vi "Egi1_Pitch_Roll_Angel_Set_Get.vi"(0 "Egi1 Roll Angle":dbl, 1 "Egi1 Roll Angle Valid":u16, 2 "message handle in 2":u64, 3 "message handle in1":u64, 5 "error in (no error)":errorcluster, 6 "Egi1 Pitch Angle Valid":u16, 8 "Egi1 Pitch Angle":dbl) -> (9 "Egi1 Roll Angle Range Message":string, 10 "Egi1 Pitch Angle Range Message":string, 11 "Egi1 Roll Angle Value NEW":u32 format="%08x", 14 "Egi1 Pitch Angle Value OLD":u32 format="%.0x", 16 "Egi1 Pitch Angle Value NEW":u32 format="%08x", 17 "Egi1 Roll Angle Value OLD":u32 format="%.0x", 19 "error out":errorcluster)   [LabVIEW 2023]
uses:
  <instrlib>/BTI429Lib/Private/Utility/Get BNR Data.vi
  <instrlib>/BTI429Lib/Private/Utility/Set BNR Data.vi
  <instrlib>/BTI429Lib/Private/Utility/Set BNR SSM.vi
  <instrlib>/BTI429Lib/BTI429LV.lvlib
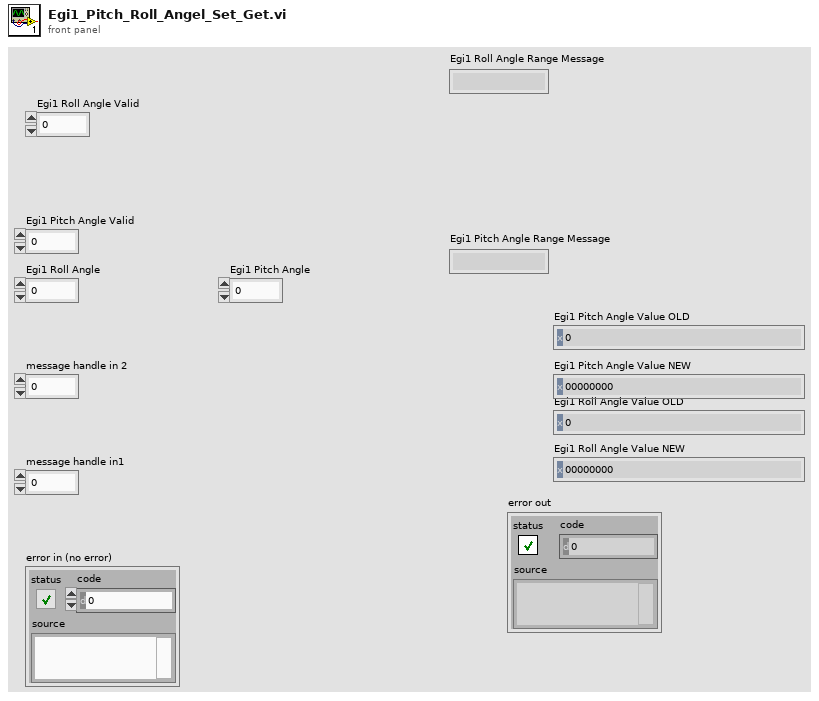
[diagram p1: front panel]
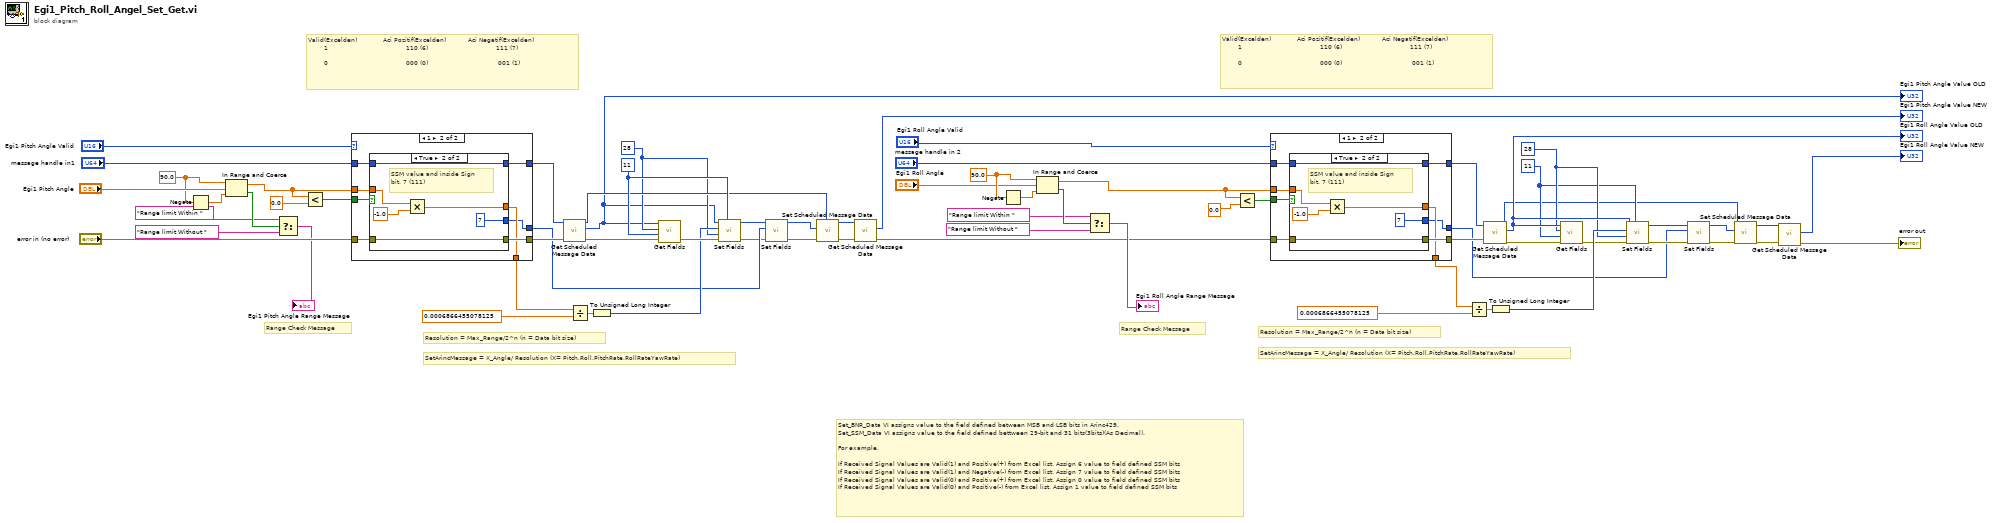
[diagram p0: block diagram]
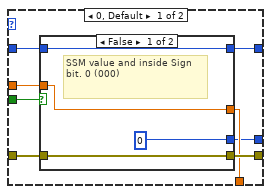
[diagram p2: hidden frame]
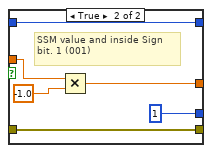
[diagram p3: hidden frame]
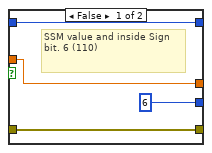
[diagram p4: hidden frame]
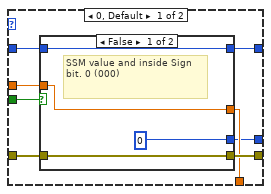
[diagram p5: hidden frame]
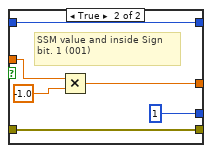
[diagram p6: hidden frame]
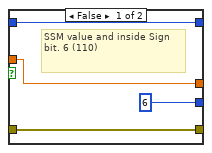
[diagram p7: hidden frame]
diagram:
  w34 = 90.0 ("upper limit")
  w40 = 90.0 ("upper limit")
  w52 = u16 28 ("most significant bit")
  w51 = u16 11 ("least significant bit")
  w23 = u16 28 ("most significant bit")
  w43 = u16 11 ("least significant bit")
  # "Range Check Message"
  # "Range Check Message"
  # "SetArincMessage = X_Angle/ Resolution (X= Pitch,Roll,PitchRate,RollRateYawRate)"
  # "Resolution = Max_Range/2^n (n = Data bit size)"
  # "SetArincMessage = X_Angle/ Resolution (X= Pitch,Roll,PitchRate,RollRateYawRate)"
  # "Resolution = Max_Range/2^n (n = Data bit size)"
  # "Set_BNR_Data VI assigns value to the field defined between MSB and LSB bits in Arinc429.\nSet_SSM_Data VI assigns value to the field defined bettween 29-bit and 31 bits(3bits)(As Decimal).\n\nFor example,\n\nIf Received Signal Values are Valid(1) and Positive(+) from Excel list. Assign 6 value to field defined SSM bits\nIf Received Signal Values are Valid(1) and Negative(-) from Excel list. Assign 7 value to field defined SSM bits\nIf Received Signal Values are Valid(0) and Positive(+) from Excel list. Assign 0 value to field defined SSM bits\nIf Received Signal Values are Valid(0) and Positive(-) from Excel list. Assign 1 value to field defined SSM bits"
  # "Valid(Excelden)             Aci Pozitif(Excelden)           Aci Negatif(Excelden) \n        1                                       110 (6)                                  111 (7)\n\n        0                                       000 (0)                                   001 (1)"
  # "Valid(Excelden)             Aci Pozitif(Excelden)           Aci Negatif(Excelden) \n        1                                       110 (6)                                  111 (7)\n\n        0                                       000 (0)                                   001 (1)"
  n1 = Negate(x=w40) -> (-x=w39:dbl)
  n2 = In Range and Coerce(upper limit=w40, x="Egi1 Pitch Angle", lower limit=w39) -> (coerced(x)=w21:dbl, In Range?=w38:bool)
  n3 = Select(t="Range limit Within ", s=w38, f="Range limit Without ") -> (s? t:f=→"Egi1 Pitch Angle Range Message":string)
  n4 = Less?(x=w21, y=0.0) -> (x < y?=w46:bool)
  n5 = case shown="1" "Egi1 Pitch Angle Valid" {
    tunnel: [w74 w93] -> w56
    tunnel: [w72 w92] -> w55
    tunnel: "error in (no error)" -> [w75 w91]
    tunnel: "message handle in1" -> [w73 w90]
    tunnel: w46 -> [w70 w89]
    tunnel: [w69 w88] -> w27
    tunnel: w21 -> [w71 w87]
    tunnel: [w68 w86] -> w19
    frame 0, Default {
      n6 = case shown="False" w70 {
        tunnel: w71 -> [w79 w81]
        tunnel: [w79 w84] -> w69
        tunnel: w73 -> [w78 w83]
        tunnel: w75 -> [w77 w82]
        tunnel: [w78 w83] -> w72
        tunnel: [w77 w82] -> w74
        tunnel: [u16 0 ("value") u16 1 ("value")] -> w68
        frame False {
          # "SSM value and inside Sign bit. 0 (000)"
        }
        frame True {
          # "SSM value and inside Sign bit. 1 (001)"
          n7 = Multiply(x=w81, y=-1.0) -> (x*y=w84:dbl)
        }
      }
    }
    frame 1 {
      n8 = case shown="True" w89 {
        tunnel: w87 -> [w97 w102]
        tunnel: [w97 w101] -> w88
        tunnel: w90 -> [w96 w100]
        tunnel: w91 -> [w95 w99]
        tunnel: [w96 w100] -> w92
        tunnel: [w95 w99] -> w93
        tunnel: [u16 6 ("value") u16 7 ("value")] -> w86
        frame False {
          # "SSM value and inside Sign bit. 6 (110)"
        }
        frame True {
          # "SSM value and inside Sign bit. 7 (111)"
          n9 = Multiply(x=w102, y=-1.0) -> (x*y=w101:dbl)
        }
      }
    }
  }
  n10 = call <instrlib>:"Get Scheduled Message Data.vi"("error in (no error)"=w56, "message handle in"=w55) -> ("error out"=w22:errorcluster, "value"=w16:u32, "message handle out"=w26:u64)  [unwired: 7 in]
  "Egi1 Pitch Angle Value OLD" <- w16
  n11 = Divide(x=w27, y=0.0006866455078125) -> (x/y=w47:dbl)
  n12 = To Unsigned Long Integer(number=w47) -> (unsigned 32bit integer=w24:u32)
  n13 = call-poly <instrlib>:"Get Fields.vi"("error in (no error)"=w22, "least significant bit"=w43, "most significant bit"=w23, "message"=w16) -> ("error out"=w25:errorcluster)  [unwired: 6 in, 1 out]
  n14 = call-poly <instrlib>:"Set Fields.vi"("least significant bit"=w43, "error in (no error)"=w25, "most significant bit"=w23, "value"=w24, "message"=w16) -> ("error out"=w14:errorcluster, "message out"=w15:u32)  [unwired: 5 in]
  n15 = call-poly <instrlib>:"Set Fields.vi"("error in (no error)"=w14, "value"=w19, "message"=w15) -> ("error out"=w18:errorcluster, "message out"=w17:u32)  [unwired: 7 in]
  n16 = call <instrlib>:"Set Scheduled Message Data.vi"("error in (no error)"=w18, "value"=w17, "message handle in"=w26) -> ("error out"=w65:errorcluster, "message handle out"=w66:u64)  [unwired: 7 in]
  n17 = call <instrlib>:"Get Scheduled Message Data.vi"("error in (no error)"=w65, "message handle in"=w66) -> ("error out"=w13:errorcluster, "value"=→"Egi1 Pitch Angle Value NEW":u32)  [unwired: 7 in, 1 out]
  n18 = Negate(x=w34) -> (-x=w33:dbl)
  n19 = In Range and Coerce(upper limit=w34, x="Egi1 Roll Angle", lower limit=w33) -> (coerced(x)=w8:dbl, In Range?=w32:bool)
  n20 = Select(t="Range limit Within ", s=w32, f="Range limit Without ") -> (s? t:f=→"Egi1 Roll Angle Range Message":string)
  n21 = Less?(x=w8, y=0.0) -> (x < y?=w7:bool)
  n22 = case shown="1" "Egi1 Roll Angle Valid" {
    tunnel: [w110 w129] -> w11
    tunnel: [w106 w128] -> w10
    tunnel: w13 -> [w111 w127]
    tunnel: "message handle in 2" -> [w105 w126]
    tunnel: w7 -> [w104 w125]
    tunnel: [w108 w124] -> w12
    tunnel: w8 -> [w109 w123]
    tunnel: [w107 w122] -> w1
    frame 0, Default {
      n23 = case shown="False" w104 {
        tunnel: w109 -> [w115 w117]
        tunnel: [w115 w120] -> w108
        tunnel: w105 -> [w114 w119]
        tunnel: w111 -> [w113 w118]
        tunnel: [w114 w119] -> w106
        tunnel: [w113 w118] -> w110
        tunnel: [u16 0 ("value") u16 1 ("value")] -> w107
        frame False {
          # "SSM value and inside Sign bit. 0 (000)"
        }
        frame True {
          # "SSM value and inside Sign bit. 1 (001)"
          n24 = Multiply(x=w117, y=-1.0) -> (x*y=w120:dbl)
        }
      }
    }
    frame 1 {
      n25 = case shown="True" w125 {
        tunnel: w123 -> [w133 w138]
        tunnel: [w133 w137] -> w124
        tunnel: w126 -> [w132 w136]
        tunnel: w127 -> [w131 w135]
        tunnel: [w132 w136] -> w128
        tunnel: [w131 w135] -> w129
        tunnel: [u16 6 ("value") u16 7 ("value")] -> w122
        frame False {
          # "SSM value and inside Sign bit. 6 (110)"
        }
        frame True {
          # "SSM value and inside Sign bit. 7 (111)"
          n26 = Multiply(x=w138, y=-1.0) -> (x*y=w137:dbl)
        }
      }
    }
  }
  n27 = Divide(x=w12, y=0.0006866455078125) -> (x/y=w59:dbl)
  n28 = call <instrlib>:"Get Scheduled Message Data.vi"("error in (no error)"=w11, "message handle in"=w10) -> ("error out"=w49:errorcluster, "value"=w61:u32, "message handle out"=w48:u64)  [unwired: 7 in]
  "Egi1 Roll Angle Value OLD" <- w61
  n29 = To Unsigned Long Integer(number=w59) -> (unsigned 32bit integer=w60:u32)
  n30 = call-poly <instrlib>:"Get Fields.vi"("error in (no error)"=w49, "least significant bit"=w51, "most significant bit"=w52, "message"=w61) -> ("error out"=w50:errorcluster)  [unwired: 6 in, 1 out]
  n31 = call-poly <instrlib>:"Set Fields.vi"("least significant bit"=w51, "error in (no error)"=w50, "most significant bit"=w52, "value"=w60, "message"=w61) -> ("error out"=w5:errorcluster, "message out"=w3:u32)  [unwired: 5 in]
  n32 = call-poly <instrlib>:"Set Fields.vi"("error in (no error)"=w5, "value"=w1, "message"=w3) -> ("error out"=w4:errorcluster, "message out"=w2:u32)  [unwired: 7 in]
  n33 = call <instrlib>:"Set Scheduled Message Data.vi"("error in (no error)"=w4, "value"=w2, "message handle in"=w48) -> ("error out"=w62:errorcluster, "message handle out"=w63:u64)  [unwired: 7 in]
  n34 = call <instrlib>:"Get Scheduled Message Data.vi"("error in (no error)"=w62, "message handle in"=w63) -> ("error out"=→"error out":errorcluster, "value"=→"Egi1 Roll Angle Value NEW":u32)  [unwired: 7 in, 1 out]
